vi "Attenuation T7.vi"(0 "Measurement":dbl caption="Measurement f" format="%.6p") -> (4 "Measurement Out":T1 caption="Measurement f" format="%.6p")   [LabVIEW 2021, in "Reusables T7.lvlib"]
uses:
  Reusables/Reusables T7.lvlib
  Measurement Result T7.ctl
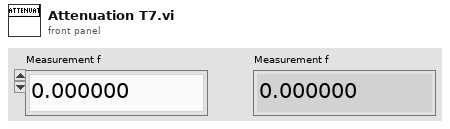
[diagram p1: front panel]
types:
  T1 = typedef "Reusables T7.lvlib/Measurement Result T7.ctl" = dbl
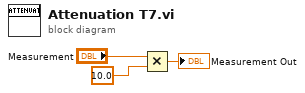
[diagram p0: block diagram]
diagram:
  n1 = Multiply(x="Measurement", y=10.0) -> (x*y=→"Measurement Out":dbl)
